vi "Set Gamma Adjust.vi"(9 "Gamma Adjust":dbl=120.0, 10 "CAN Offset":u32=160 format="%x", 11 "CANTXQueueIn":T1) -> (3 "CANTXQueueOut":T1)   [LabVIEW 2014]
uses:
  TX Library/CAN Message Queue.ctl
  TX Library/CAN Message.ctl
  TX Library/Transmit CAN.vi
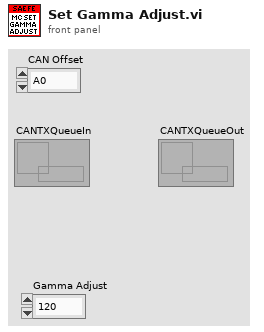
[diagram p1: front panel]
types:
  T1 = typedef "CAN Message Queue.ctl" = refnum<k33>
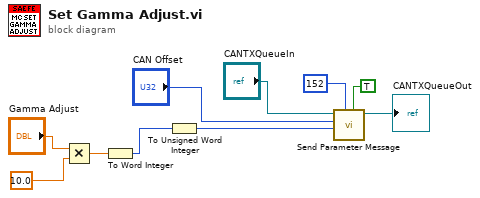
[diagram p0: block diagram]
diagram:
  n1 = Multiply(x="Gamma Adjust", y=10.0) -> (x*y=w6:dbl)
  n2 = To Word Integer(number=w6) -> (16bit integer=w4:i16)
  n3 = To Unsigned Word Integer(number=w4) -> (unsigned 16bit integer=w3:u16)
  n4 = call "Send Parameter Message.vi"("Write?"=TRUE, "Param Address"=i16 152, "Data"=w3, "CAN Offset"="CAN Offset", "CANTXQueueIn"="CANTXQueueIn") -> ("CANTXQueueOut"=→"CANTXQueueOut":T1)  [unwired: 6 in]
